vi "test-new-clock-benchmark.vi"() -> ()   [LabVIEW 2020]
uses:
  <vilib>/Rock Robotics/WPI/ThirdParty/JAS_Junk/TrajLib/VI/Util_GetTime_U32.vi
  <vilib>/Rock Robotics/SystemInterfaces/Utilities/FPGA_UtilitiesRead LocalTime.vi
  <vilib>/Rock Robotics/WPI/ThirdParty/JAS_Junk/TrajLib/VI/Util_GetTime_U64.vi
  <vilib>/Rock Robotics/WPI/ThirdParty/JAS_Junk/TrajLib/Trajectory_Library.lvlib
panel:
  out "Avg Loop US":dbl
  out "Per Loop US":dbl
  out "Error Count":i32
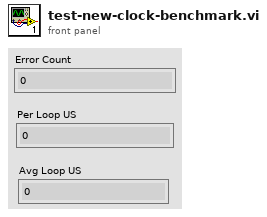
[diagram p1: front panel]
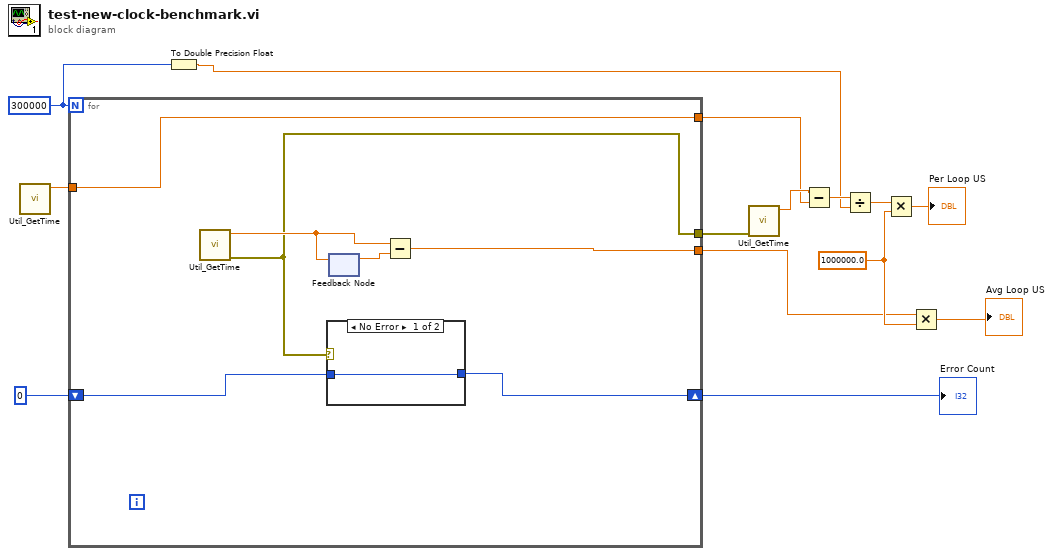
[diagram p0: block diagram]
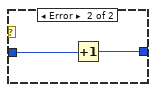
[diagram p2: hidden frame]
diagram:
  w3 = 1000000.0 ("y")
  w11 = 300000
  n1 = call <vilib>:"Util_GetTime.vi"() -> ("FPGA_Time_Seconds"=w14:dbl)  [unwired: 9 in, 2 out]
  n2 = for {
    N: w11 -> [_]
    tunnel: w14 -> [w16]
    shift-right: [w18] -> w7
    shift-left: 0 -> [w21]
    tunnel: [w15] -> w2
    tunnel: [w17] -> w12
    tunnel: [w16] -> w4
    n3 = call <vilib>:"Util_GetTime.vi"() -> ("error out"=w17:errorcluster, "FPGA_Time_Seconds"=w20:dbl)  [unwired: 9 in, 1 out]
    n4 = case shown="No Error" w17 {
      tunnel: [w22 w24] -> w18
      tunnel: w21 -> [w22 w23]
      frame No Error {
      }
      frame Error {
        n5 = Increment(x=w23) -> (x+1=w24:i32)
      }
    }
    n6 = feedback-in #1(w20) -> ()
    n7 = feedback #1() -> (w19:dbl)  [unwired: 1 in]
    n8 = Subtract(x=w20, y=w19) -> (x-y=w15:dbl)
  }
  "Error Count" <- w7
  n9 = To Double Precision Float(number=w11) -> (double precision float=w9:dbl)
  n10 = call <vilib>:"Util_GetTime.vi"("error in (no error)"=w12) -> ("FPGA_Time_Seconds"=w5:dbl)  [unwired: 8 in, 2 out]
  n11 = Subtract(x=w5, y=w4) -> (x-y=w10:dbl)
  n12 = Divide(x=w10, y=w9) -> (x/y=w8:dbl)
  n13 = Multiply(x=w8, y=w3) -> (x*y=→"Per Loop US":dbl)
  n14 = Multiply(x=w2, y=w3) -> (x*y=→"Avg Loop US":dbl)
